vi "判定2.vi"(6 "显示超限点":bool, 7 "方式":enum16{"清除曲线", "显示判定框", "判定曲线"}(ring), 8 "错误输入":errorcluster, 10 "曲线判定条件":T2(array[cluster]), 11 "曲线引用":refnum<vi>) -> (0 "错误输出":errorcluster, 2 "曲线判定结果":T1(array[cluster]), 3 "曲线引用输出":refnum<vi>)   [LabVIEW 2017]
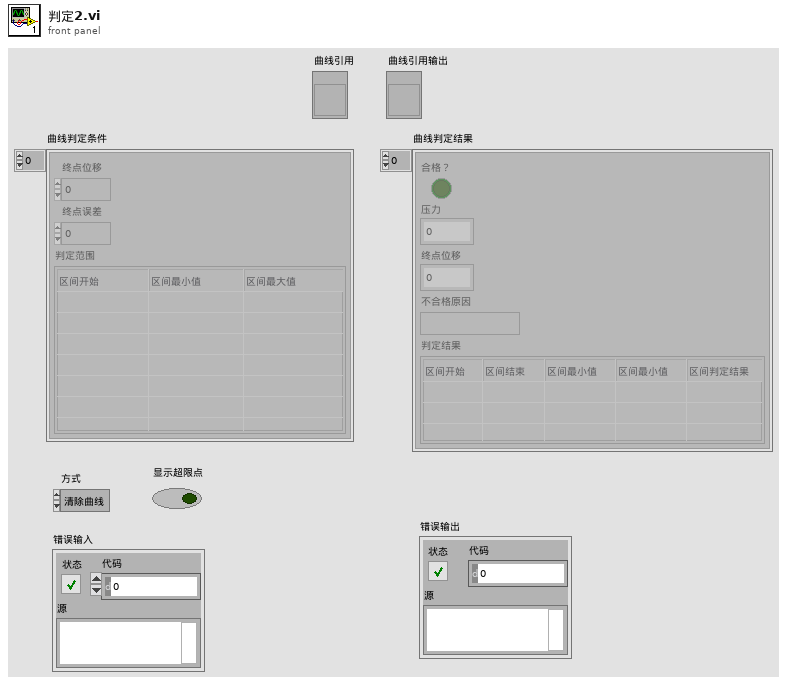
[diagram p1: front panel]
types:
  T1 = cluster{"合格？":bool, "压力":dbl, "终点位移":dbl, "不合格原因":string, "判定结果":string[][]}[]
  T2 = cluster{"终点位移":dbl, "终点误差":dbl, "判定范围":string[][]}[]
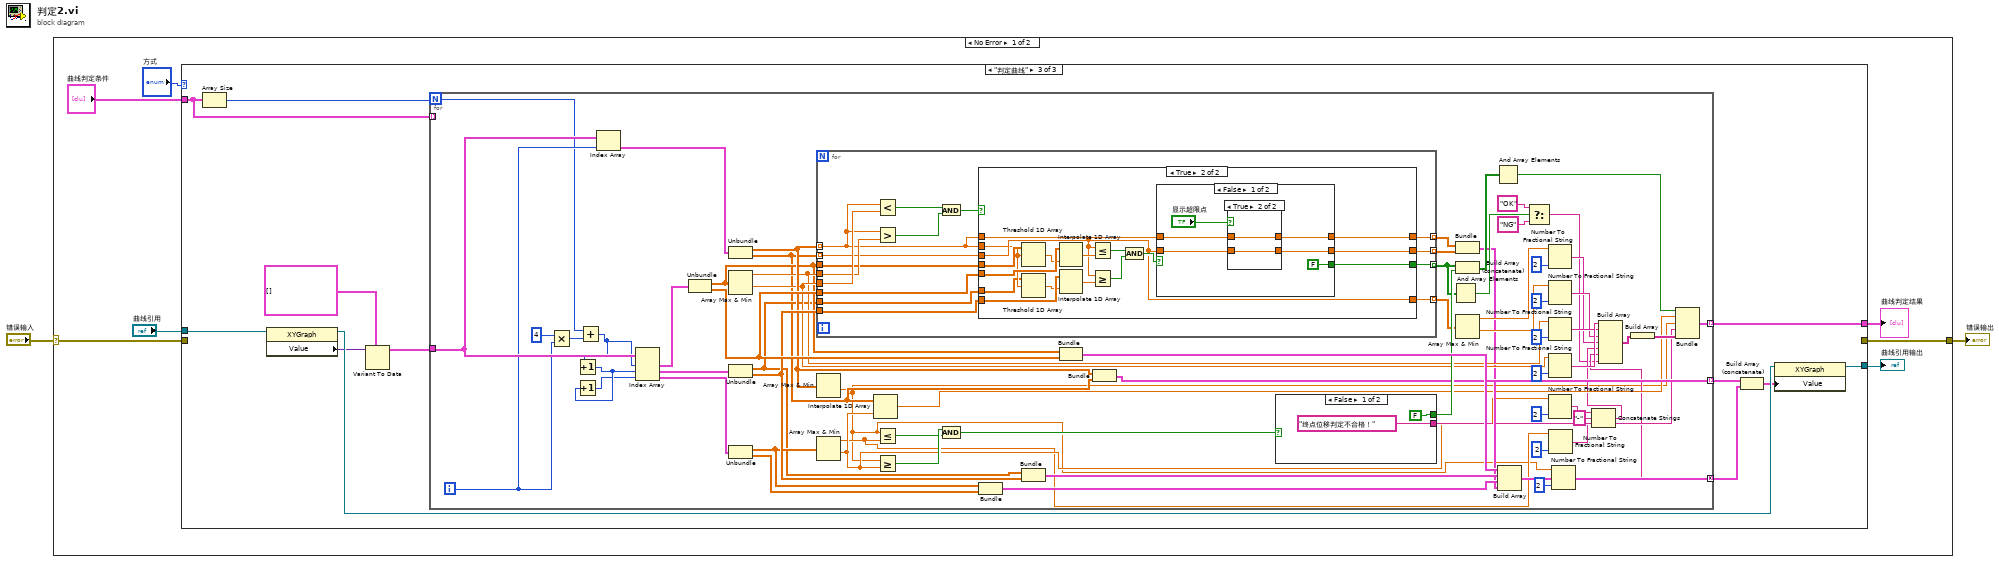
[diagram p0: block diagram]
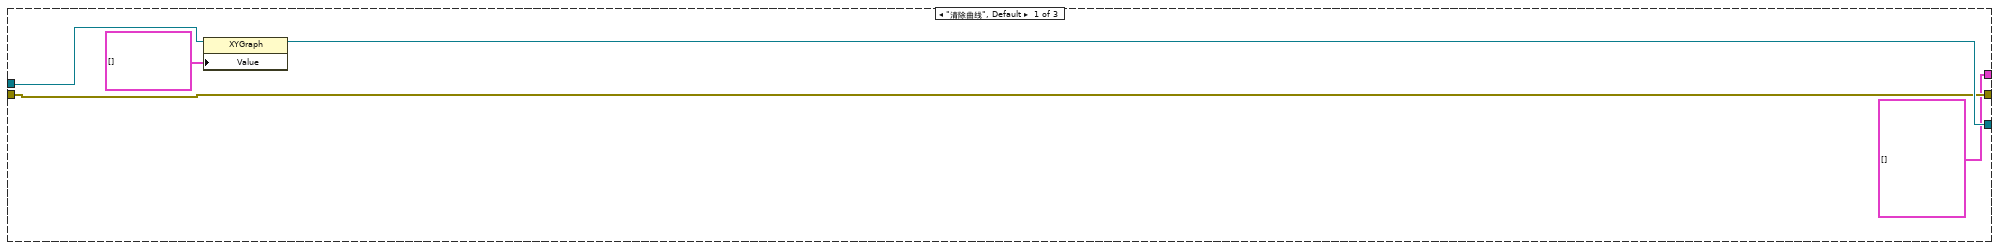
[diagram p2: hidden frame]
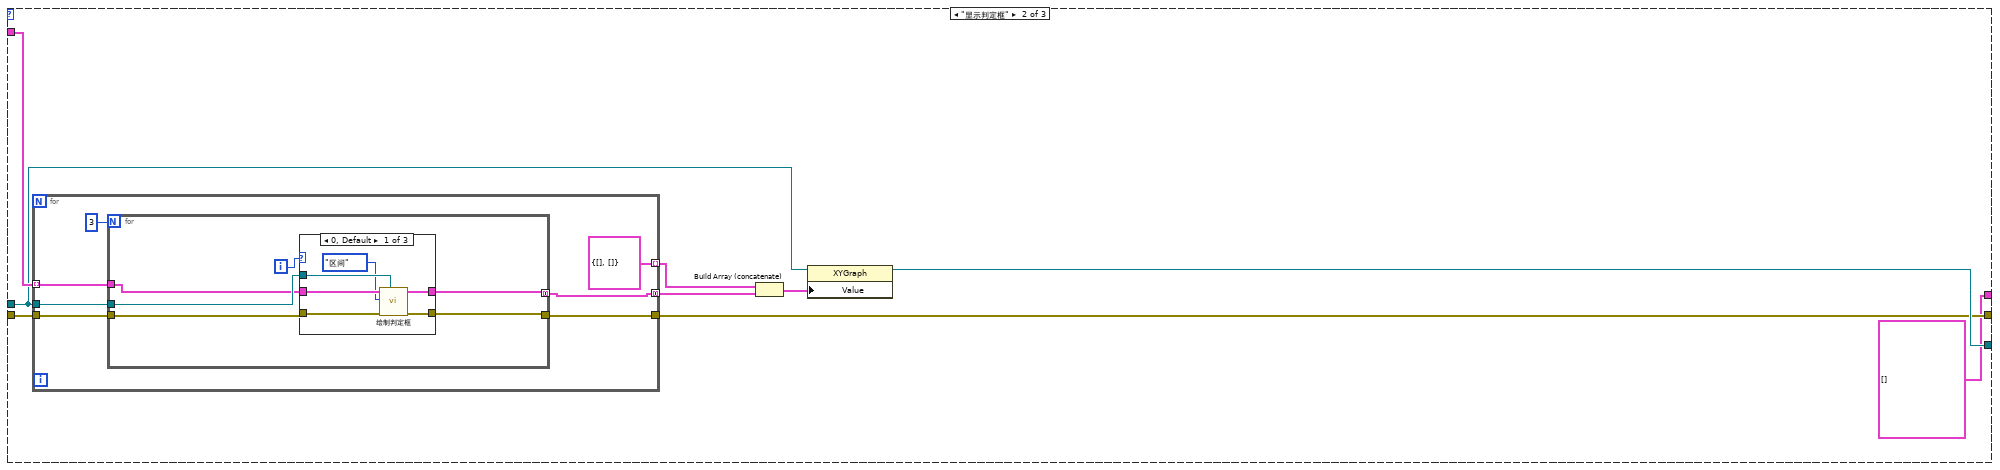
[diagram p3: hidden frame]
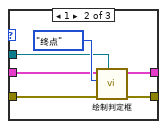
[diagram p4: hidden frame]
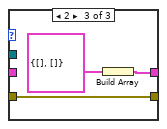
[diagram p5: hidden frame]
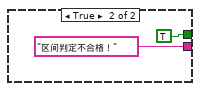
[diagram p6: hidden frame]
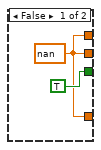
[diagram p7: hidden frame]
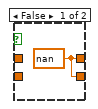
[diagram p8: hidden frame]
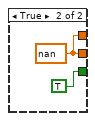
[diagram p9: hidden frame]
diagram:
  n1 = case shown="No Error" "错误输入" {
    selector: "错误输入" -> [w5 w181]
    tunnel: [w4 w181] -> w1
    frame No Error {
      n2 = case shown="\"判定曲线\"" "方式" {
        tunnel: "曲线引用" -> [w14 w18 w63]
        tunnel: [w13 w23 w61] -> w7
        tunnel: "曲线判定条件" -> [_ w22 w55]
        tunnel: w5 -> [w11 w17 _]
        tunnel: [w11 w16 _] -> w4
        tunnel: [cluster{bool, dbl, dbl, string, string[][]}[] [] cluster{bool, dbl, dbl, string, string[][]}[] [] w52] -> w3
        frame "清除曲线", Default {
          n3 = property class="XYGraph"(reference=w14, "Value"=cluster{dbl[], dbl[]}[] []) -> (reference out=w13:refnum<vi>)  [unwired: 1 in, 1 out]
        }
        frame "显示判定框" {
          n4 = for {
            tunnel: [w30] -> w21 mode=concatenating
            tunnel: w22 -> [w26] mode=indexing
            tunnel: [cluster{dbl[], dbl[]} {[], []}] -> w20 mode=indexing
            tunnel: w18 -> [w27]
            tunnel: w17 -> [w25]
            tunnel: [w24] -> w16
            n5 = for {
              N: 3 -> [_]
              tunnel: [w35] -> w30 mode=concatenating
              tunnel: w27 -> [w34]
              tunnel: w26 -> [w33]
              tunnel: w25 -> [w32]
              tunnel: [w31] -> w24
              i -> [w36]
              n6 = case shown="0, Default" w36 {
                tunnel: [w37 w43 w49] -> w35
                tunnel: w34 -> [w42 w47 _]
                tunnel: w33 -> [w41 w44 _]
                tunnel: w32 -> [w39 w46 w51]
                tunnel: [w38 w45 w51] -> w31
                frame 0, Default {
                  n7 = call "绘制判定框.vi"("曲线引用"=w42, "error in (no error)"=w39, "判定框类型"=enum16{"区间", "终点"}."区间", "曲线判定条件"=w41) -> ("error out"=w38:errorcluster, "判定框"=w37:cluster{"横坐标":dbl[], "纵坐标":dbl[]}[])  [unwired: 6 in]
                }
                frame 1 {
                  n8 = call "绘制判定框.vi"("曲线引用"=w47, "error in (no error)"=w46, "判定框类型"=enum16{"区间", "终点"}."终点", "曲线判定条件"=w44) -> ("error out"=w45:errorcluster, "判定框"=w43:cluster{"横坐标":dbl[], "纵坐标":dbl[]}[])  [unwired: 6 in]
                }
                frame 2 {
                  n9 = Build Array(cluster{dbl[], dbl[]} {[], []}) -> (w49:cluster{dbl[], dbl[]}[])
                }
              }
            }
          }
          n10 = Build Array (concatenate)(w20, w21) -> (w19:cluster{"横坐标":dbl[], "纵坐标":dbl[]}[])
          n11 = property class="XYGraph"(reference=w18, "Value"=w19) -> (reference out=w23:refnum<vi>)  [unwired: 1 in, 1 out]
        }
        frame "判定曲线" {
          n12 = Array Size(array=w55) -> (size(s)=w57:i32)
          n13 = property class="XYGraph"(reference=w63) -> (reference out=w62:refnum<vi>, "Value"=w60:variant)  [unwired: 1 in, 1 out]
          n14 = Variant To Data(type=cluster{dbl[], dbl[]}[] [], Variant=w60) -> (data=w58:cluster{dbl[], dbl[]}[])  [unwired: 1 in, 1 out]
          n15 = for {
            N: w57 -> [w68]
            tunnel: w58 -> [w74]
            tunnel: [w125] -> w53 mode=concatenating
            tunnel: w55 -> [_] mode=indexing
            tunnel: [w103] -> w54 mode=indexing
            tunnel: [w91] -> w52 mode=indexing
            i -> [w70]
            n16 = Multiply(x=4, y=w70) -> (x*y=w67:i32)
            n17 = Add(x=w68, y=w67) -> (x+y=w66:i32)
            n18 = Increment(x=w66) -> (x+1=w72:i32)
            n19 = Increment(x=w72) -> (x+1=w71:i32)
            n20 = Index Array(array=w74, index=w70) -> (element=w73:cluster{dbl[], dbl[]})
            n21 = Index Array(array=w74, index #1=w66, index #2=w72, index #3=w71) -> (element #1=w131:cluster{dbl[], dbl[]}, element #2=w130:cluster{dbl[], dbl[]}, element #3=w102:cluster{dbl[], dbl[]})
            n22 = Unbundle(w131) -> (w98:dbl[], w129:dbl[])
            n23 = Unbundle(w73) -> (w124:dbl[], w65:dbl[])
            n24 = Array Max & Min(array=w98) -> (max value=w117:dbl, min value=w118:dbl)  [unwired: 2 out]
            n25 = Unbundle(w130) -> (w90:dbl[], w128:dbl[])
            n26 = Unbundle(w102) -> (w101:dbl[], w100:dbl[])
            n27 = for {
              tunnel: w124 -> [w139] mode=indexing
              tunnel: w65 -> [w142] mode=indexing
              tunnel: w129 -> [w145]
              tunnel: w117 -> [w149]
              tunnel: w118 -> [w150]
              tunnel: w128 -> [w144]
              tunnel: [w143] -> w114 mode=indexing
              tunnel: [w141] -> w119 mode=indexing
              tunnel: w98 -> [w140]
              tunnel: [w138] -> w97 mode=indexing
              tunnel: [w137] -> w95 mode=indexing
              tunnel: w90 -> [w136]
              n28 = Less?(x=w139, y=w150) -> (x < y?=w147:bool)
              n29 = Greater?(x=w139, y=w149) -> (0:w148:bool)
              n30 = And(x=w147, y=w148) -> (x .and. y?=w146:bool)
              n31 = case shown="True" w146 {
                tunnel: w145 -> [_ w169]
                tunnel: w139 -> [_ w161]
                tunnel: w142 -> [_ w160]
                tunnel: w144 -> [_ w168]
                tunnel: [TRUE w162] -> w143
                tunnel: [w151 w160] -> w141
                tunnel: w140 -> [_ w159]
                tunnel: w139 -> [_ w155]
                tunnel: [w151 w157] -> w138
                tunnel: [w151 w156] -> w137
                tunnel: w136 -> [_ w154]
                frame False {
                  w151 = nan ("New Element/Subarray")
                }
                frame True {
                  n32 = Threshold 1D Array(2:w155, 3:w159) -> (0:w158:dbl)  [unwired: 1 in]
                  n33 = Threshold 1D Array(2:w155, 3:w154) -> (0:w153:dbl)  [unwired: 1 in]
                  n34 = Interpolate 1D Array(1:w158, 2:w169) -> (0:w167:dbl)
                  n35 = Interpolate 1D Array(1:w153, 2:w168) -> (0:w166:dbl)
                  n36 = Less Or Equal?(x=w160, y=w167) -> (x <= y?=w164:bool)
                  n37 = Greater Or Equal?(x=w160, y=w166) -> (x >= y?=w165:bool)
                  n38 = And(x=w164, y=w165) -> (x .and. y?=w163:bool)
                  n39 = case shown="False" w163 {
                    tunnel: [FALSE TRUE] -> w162
                    tunnel: w161 -> [w173 _]
                    tunnel: w160 -> [w172 _]
                    tunnel: [w171 w179] -> w157
                    tunnel: [w170 w179] -> w156
                    frame False {
                      n40 = case shown="True" "显示超限点" {
                        tunnel: w173 -> [_ w178]
                        tunnel: w172 -> [_ w177]
                        tunnel: [w176 w178] -> w171
                        tunnel: [w176 w177] -> w170
                        frame False {
                          w176 = nan ("New Element/Subarray")
                        }
                        frame True {
                        }
                      }
                    }
                    frame True {
                      w179 = nan ("New Element/Subarray")
                    }
                  }
                }
              }
            }
            n41 = Array Max & Min(array=w124) -> (min value=w64:dbl)  [unwired: 3 out]
            n42 = Array Max & Min(array=w101) -> (max value=w77:dbl, min value=w82:dbl)  [unwired: 2 out]
            n43 = Interpolate 1D Array(1:w82, 2:w65) -> (0:w92:dbl)
            n44 = Less Or Equal?(x=w64, y=w77) -> (x <= y?=w122:bool)
            n45 = Greater Or Equal?(x=w64, y=w82) -> (x >= y?=w123:bool)
            n46 = And(x=w123, y=w122) -> (x .and. y?=w121:bool)
            n47 = Bundle(w101, w100) -> (w99:cluster{dbl[], dbl[]})  [unwired: 1 in]
            n48 = Bundle(w90, w128) -> (w126:cluster{dbl[], dbl[]})  [unwired: 1 in]
            n49 = Bundle(w98, w129) -> (w127:cluster{dbl[], dbl[]})  [unwired: 1 in]
            n50 = Bundle(w124, w65) -> (w103:cluster{dbl[], dbl[]})  [unwired: 1 in]
            n51 = case shown="False" w121 {
              tunnel: [FALSE TRUE] -> w120
              tunnel: ["终点位移判定不合格！" "区间判定不合格！"] -> w93
              frame False {
              }
              frame True {
              }
            }
            n52 = And Array Elements(Boolean array=w114) -> (logical AND=w113:bool)
            n53 = Bundle(w97, w95) -> (w96:cluster{dbl[], dbl[]})  [unwired: 1 in]
            n54 = Build Array (concatenate)(w114, w120) -> (w105:bool[])
            n55 = Array Max & Min(array=w119) -> (max value=w115:dbl, min value=w116:dbl)  [unwired: 2 out]
            n56 = And Array Elements(Boolean array=w105) -> (logical AND=w104:bool)
            n57 = Build Array(w127, w126, w99, w96) -> (w125:cluster{dbl[], dbl[]}[])
            n58 = Select(t="OK", s=w113, f="NG") -> (s? t:f=w75:string)
            n59 = Number To Fractional String(number=w115, precision (6)=i16 2 ("精度(6)")) -> (F-format string=w107:string)  [unwired: 2 in]
            n60 = Number To Fractional String(number=w116, precision (6)=i16 2 ("精度(6)")) -> (F-format string=w108:string)  [unwired: 2 in]
            n61 = Number To Fractional String(number=w117, precision (6)=i16 2 ("精度(6)")) -> (F-format string=w109:string)  [unwired: 2 in]
            n62 = Number To Fractional String(number=w118, precision (6)=i16 2 ("精度(6)")) -> (F-format string=w110:string)  [unwired: 2 in]
            n63 = Number To Fractional String(number=w82, precision (6)=i16 2 ("精度(6)")) -> (F-format string=w81:string)  [unwired: 2 in]
            n64 = Number To Fractional String(number=w77, precision (6)=i16 2 ("精度(6)")) -> (F-format string=w79:string)  [unwired: 2 in]
            n65 = Number To Fractional String(number=w64, precision (6)=i16 2 ("精度(6)")) -> (F-format string=w76:string)  [unwired: 2 in]
            n66 = Concatenate Strings(w81, "-" ("字符串"), w79) -> (w78:string)
            n67 = Build Array(w110, w109, w108, w107, w78, w76, w75) -> (w106:string[])
            n68 = Build Array(w106) -> (w94:string[][])
            n69 = Bundle(w104, w92, w64, w93, w94) -> (w91:cluster{bool, dbl, dbl, string, string[][]})  [unwired: 1 in]
          }
          n70 = Build Array (concatenate)(w54, w53) -> (w56:cluster{dbl[], dbl[]}[])
          n71 = property class="XYGraph"(reference=w62, "Value"=w56) -> (reference out=w61:refnum<vi>)  [unwired: 1 in, 1 out]
        }
      }
      "曲线引用输出" <- w7
      "曲线判定结果" <- w3
    }
    frame Error {
    }
  }
  "错误输出" <- w1
